vi "Configure_MyCamera.vi"(4 "Camera Error In":errorcluster, 5 "ExposureTime (ms)":dbl=20.0, 6 "Camera Type":u16(ring) items=["AVT Manta", "Hamamatsu Orca", "Photonfocus GigE"], 7 "Camera Session In":T1 caption="Session Out") -> (0 "Camera Error Out":errorcluster, 3 "Camera Session Out":T1 caption="Session Out")   [LabVIEW 2014]
doc: "Allows the user to focus the camera on the sample"
uses:
  <vilib>/userdefined/High Color/IMAQdx.ctl
  Widefield_globals.vi
  <resource>/objmgr/imaqdx.rc
  <vilib>/vision/driver/NI_Vision_Acquisition_Software.lvlib
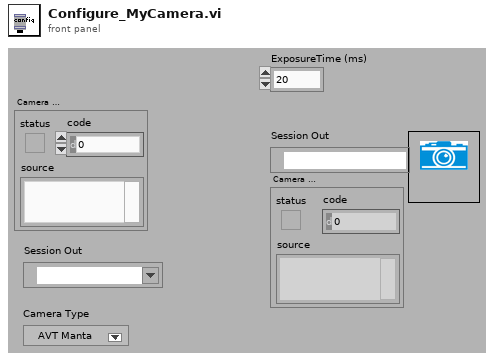
[diagram p1: front panel]
types:
  T1 = typedef "IMAQdx.ctl" = refnum<k21>
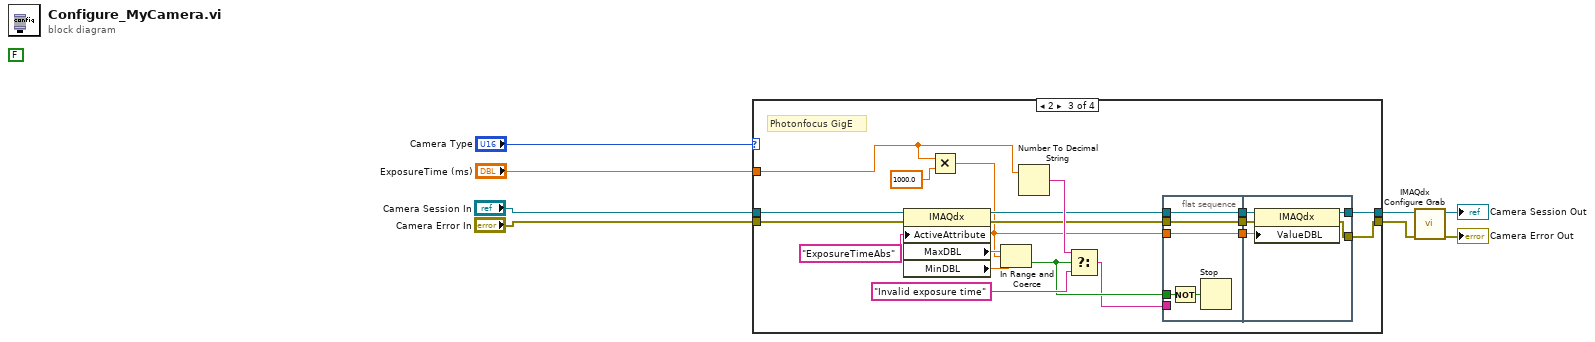
[diagram p0: block diagram]
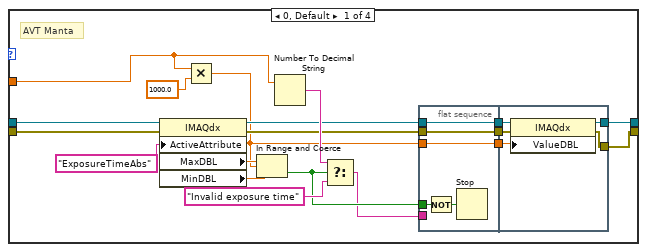
[diagram p2: hidden frame]
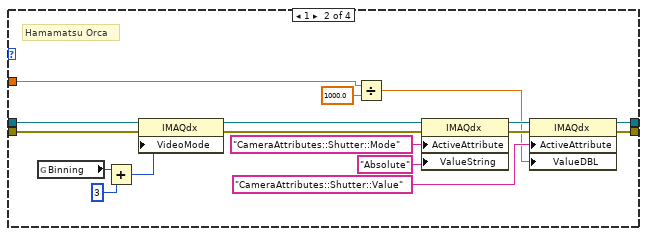
[diagram p3: hidden frame]
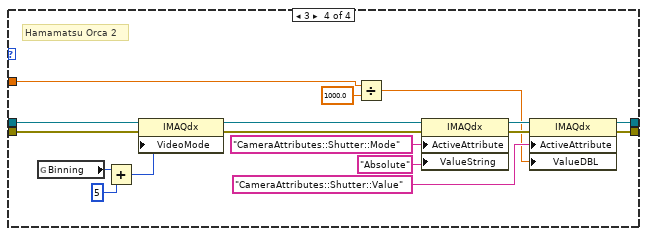
[diagram p4: hidden frame]
diagram:
  (unwired) FALSE ("Snap!")
  n1 = case shown="2" "Camera Type" {
    tunnel: [w12 w54 w58 w100] -> w8
    tunnel: [w13 w53 w59 w99] -> w7
    tunnel: "ExposureTime (ms)" -> [w9 w50 w55 w96]
    tunnel: "Camera Session In" -> [w11 w39 w57 w85]
    tunnel: "Camera Error In" -> [w10 w38 w56 w84]
    frame 0, Default {
      # "AVT Manta"
      n2 = property class="IMAQdx"(reference=w11, error in=w10, "ActiveAttribute"="ExposureTimeAbs" ("Camera Attribute")) -> (reference out=w18:T1, error out=w17:errorcluster, "MaxDBL"=w23:dbl, "MinDBL"=w15:dbl)
      n3 = Multiply(x=w9, y=1000.0) -> (x*y=w16:dbl)
      n4 = In Range and Coerce(upper limit=w23, x=w16, lower limit=w15) -> (In Range?=w19:bool)  [unwired: 1 out]
      n5 = Number To Decimal String(number=w9) -> (decimal integer string=w20:string)  [unwired: 1 out]
      n6 = Select(t=w20, s=w19, f="Invalid exposure time") -> (s? t:f=w14:string)
      n7 = flat-sequence {
        tunnel: w14 -> [_]
        tunnel: w19 -> [w31]
        tunnel: w18 -> [w29]
        tunnel: w17 -> [w30]
        tunnel: [w30] -> w27
        tunnel: [w29] -> w26
        tunnel: [w28] -> w25
        tunnel: w16 -> [w28]
        tunnel: w27 -> [w36]
        tunnel: w26 -> [w37]
        tunnel: w25 -> [w35]
        tunnel: [w34] -> w13
        tunnel: [w33] -> w12
        frame #0 {
          n8 = Not(x=w31) -> (.not. x?=w32:bool)
          n9 = Stop(stop? (T)=w32) -> ()
        }
        frame #1 {
          n10 = property class="IMAQdx"(reference=w37, error in=w36, "ValueDBL"=w35) -> (reference out=w34:T1, error out=w33:errorcluster)
        }
      }
    }
    frame 1 {
      # "Hamamatsu Orca"
      n11 = global read "Widefield_globals.vi" "Binning"() -> (w40:u16)
      n12 = Add(x=w40, y=u16 3) -> (x+y=w42:u16)
      n13 = property class="IMAQdx"(reference=w39, error in=w38, "VideoMode"=w42) -> (reference out=w44:T1, error out=w43:errorcluster)
      n14 = Divide(x=w50, y=1000.0) -> (x/y=w45:dbl)
      n15 = property class="IMAQdx"(reference=w44, error in=w43, "ActiveAttribute"="CameraAttributes::Shutter::Mode", "ValueString"="Absolute") -> (reference out=w47:T1, error out=w48:errorcluster)
      n16 = property class="IMAQdx"(reference=w47, error in=w48, "ActiveAttribute"="CameraAttributes::Shutter::Value", "ValueDBL"=w45) -> (reference out=w53:T1, error out=w54:errorcluster)
    }
    frame 2 {
      # "Photonfocus GigE"
      n17 = property class="IMAQdx"(reference=w57, error in=w56, "ActiveAttribute"="ExposureTimeAbs" ("Camera Attribute")) -> (reference out=w64:T1, error out=w63:errorcluster, "MaxDBL"=w69:dbl, "MinDBL"=w61:dbl)
      n18 = Multiply(x=w55, y=1000.0) -> (x*y=w62:dbl)
      n19 = In Range and Coerce(upper limit=w69, x=w62, lower limit=w61) -> (In Range?=w65:bool)  [unwired: 1 out]
      n20 = Number To Decimal String(number=w55) -> (decimal integer string=w66:string)  [unwired: 1 out]
      n21 = Select(t=w66, s=w65, f="Invalid exposure time") -> (s? t:f=w60:string)
      n22 = flat-sequence {
        tunnel: w60 -> [_]
        tunnel: w65 -> [w77]
        tunnel: w64 -> [w75]
        tunnel: w63 -> [w76]
        tunnel: [w76] -> w73
        tunnel: [w75] -> w72
        tunnel: [w74] -> w71
        tunnel: w62 -> [w74]
        tunnel: w73 -> [w82]
        tunnel: w72 -> [w83]
        tunnel: w71 -> [w81]
        tunnel: [w80] -> w59
        tunnel: [w79] -> w58
        frame #0 {
          n23 = Not(x=w77) -> (.not. x?=w78:bool)
          n24 = Stop(stop? (T)=w78) -> ()
        }
        frame #1 {
          n25 = property class="IMAQdx"(reference=w83, error in=w82, "ValueDBL"=w81) -> (reference out=w80:T1, error out=w79:errorcluster)
        }
      }
    }
    frame 3 {
      # "Hamamatsu Orca 2"
      n26 = global read "Widefield_globals.vi" "Binning"() -> (w86:u16)
      n27 = Add(x=w86, y=u16 5) -> (x+y=w88:u16)
      n28 = property class="IMAQdx"(reference=w85, error in=w84, "VideoMode"=w88) -> (reference out=w90:T1, error out=w89:errorcluster)
      n29 = Divide(x=w96, y=1000.0) -> (x/y=w91:dbl)
      n30 = property class="IMAQdx"(reference=w90, error in=w89, "ActiveAttribute"="CameraAttributes::Shutter::Mode", "ValueString"="Absolute") -> (reference out=w93:T1, error out=w94:errorcluster)
      n31 = property class="IMAQdx"(reference=w93, error in=w94, "ActiveAttribute"="CameraAttributes::Shutter::Value", "ValueDBL"=w91) -> (reference out=w99:T1, error out=w100:errorcluster)
    }
  }
  n32 = call <vilib>:"IMAQdx Configure Grab.vi"("error in"=w8, "Session In"=w7) -> ("error out"=→"Camera Error Out":errorcluster, "Session Out"=→"Camera Session Out":T1)  [unwired: 8 out]
